vi "Qudi_multicolour_scan.vi"(3 "N Z positions":i32) -> ()   [LabVIEW 2015]
uses:
  <vilib>/rvi/Emulation/niFpgaGetClockAttributes.vi
  <vilib>/rvi/Emulation/niFpgaSctlEmulationGetInTimedLoop.vi
  <vilib>/rvi/Emulation/niFpgaEmulationReportErrorSimple.vi
  <vilib>/rvi/eio/common/nirviEmuTemplateMethod_errors.vi
  <vilib>/rvi/Emulation/niFpgaProcessEmulError.vi
  <vilib>/rvi/Emulation/niFpgaCriticalErrorInLSC.vi
  <vilib>/eio/EIONode/EIONode.xnode
panel:
  in  "exposure_time_ms":u16
  in  "stop":bool
  out "n cycles":i32
  out "Images acquired":i32
  in  "Laser lines":i32[](array[numeric])=[0, 0, 0, 0, 0, 0, 0, 0, 0, 0]
  in  "N laser lines":i32
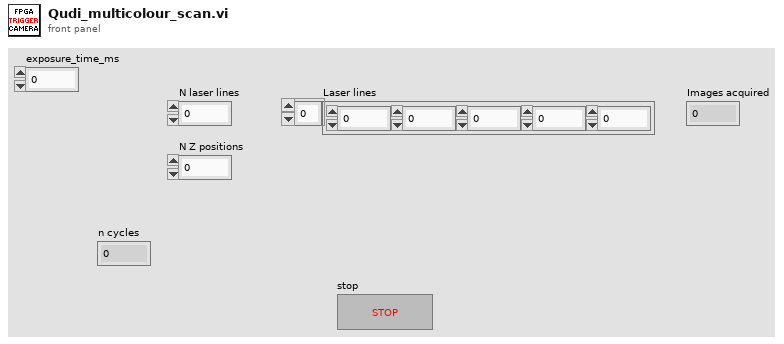
[diagram p1: front panel]
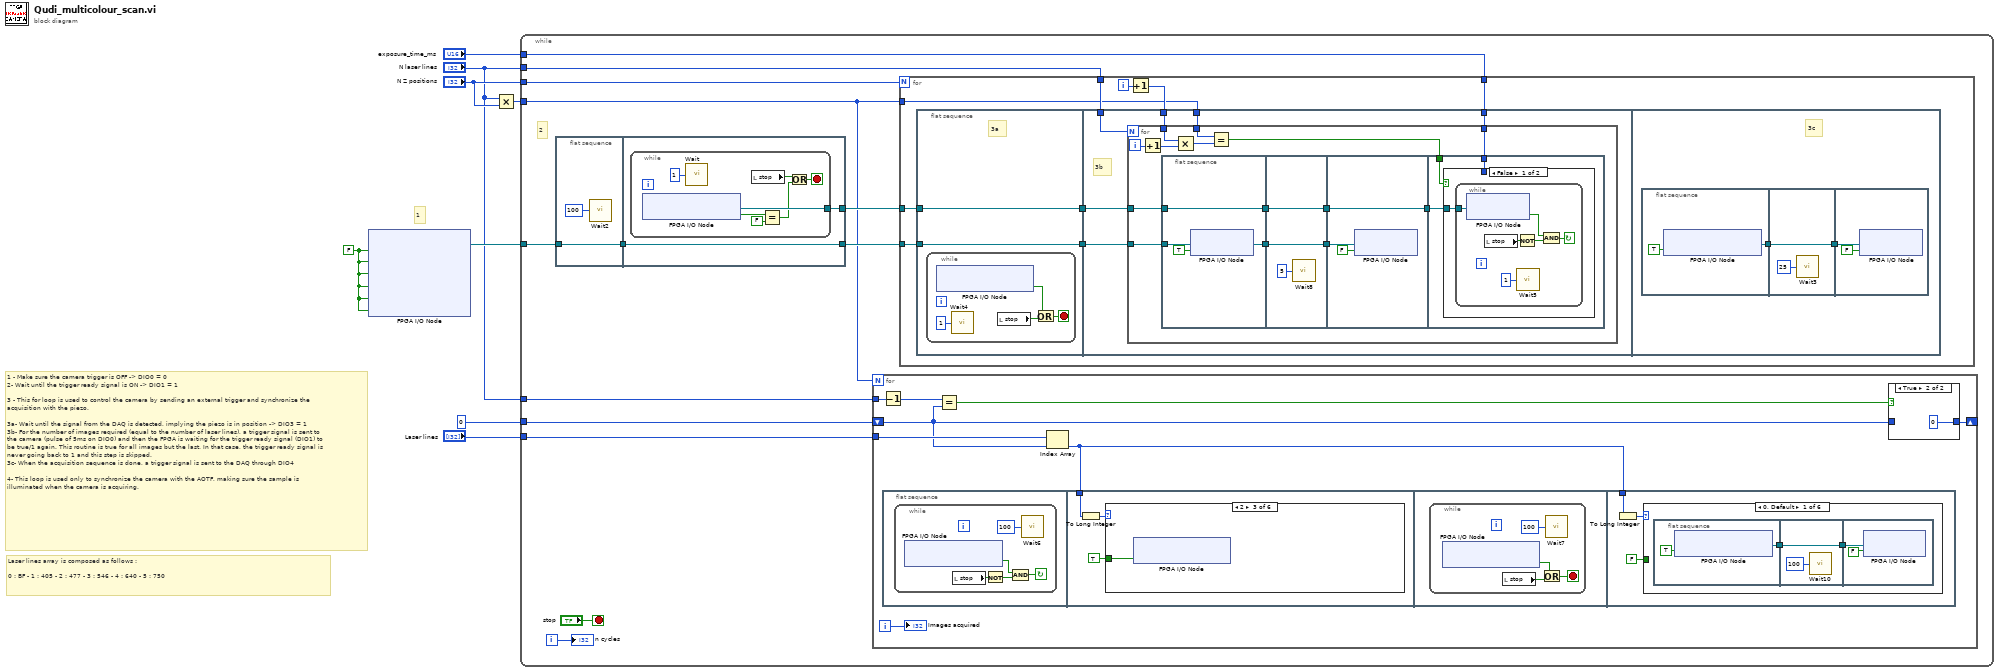
[diagram p0: block diagram]
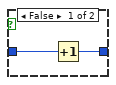
[diagram p2: hidden frame]
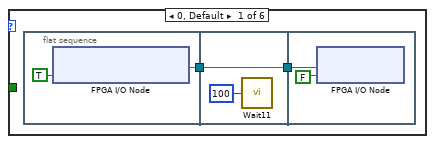
[diagram p3: hidden frame]
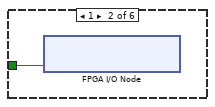
[diagram p4: hidden frame]
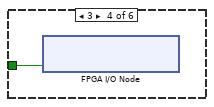
[diagram p5: hidden frame]
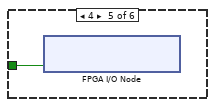
[diagram p6: hidden frame]
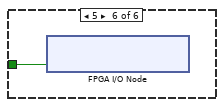
[diagram p7: hidden frame]
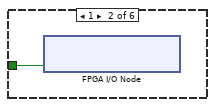
[diagram p8: hidden frame]
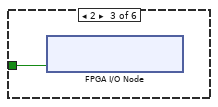
[diagram p9: hidden frame]
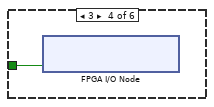
[diagram p10: hidden frame]
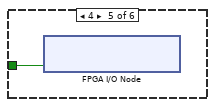
[diagram p11: hidden frame]
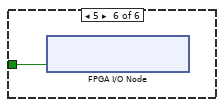
[diagram p12: hidden frame]
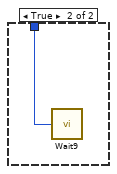
[diagram p13: hidden frame]
diagram:
  w1 = FALSE ("Connector0/DIO0")
  # "Laser lines array is composed as follows :\n\n0 : BF - 1 : 405 - 2 : 477 - 3 : 546 - 4 : 640 - 5 : 750"
  # "1"
  # "1 - Make sure the camera trigger is OFF -> DIO0 = 0\n2- Wait until the trigger ready signal is ON -> DIO1 = 1\n\n3 - This for loop is used to control the camera by sending an external trigger and synchronize the acquisition with the piezo.\n\n3a- Wait until the signal from the DAQ is detected, implying the piezo is in position -> DIO3 = 1 \n3b- For the number of images required (equal to the number of laser lines), a trigger signal is sent to the camera (pulse of 5ms on DIO0) and then the FPGA is waiting for the trigger ready signal (DIO1) to be true/1 again. This routine is true for all images but the last. In that case, the trigger ready signal is never going back to 1 and this step is skipped. \n3c- When the acquisition sequence is done, a trigger signal is sent to the DAQ through DIO4\n\n4- This loop is used only to synchronize the camera with the AOTF, making sure the sample is illuminated when the camera is acquiring."
  n1 = xnode "FPGA I/O Node"("Connector0/DIO0"=w1, "Connector0/DIO6"=w1, "Connector0/DIO7"=w1, "Connector0/DIO8"=w1, "Connector0/DIO9"=w1, "Connector0/DIO10"=w1) -> ("FPGA I/O Out"=w8:refnum<k21>)  [unwired: 6 in, 5 out]
  n2 = Multiply(x="N laser lines", y="N Z positions") -> (x*y=w4:i32)
  n3 = while {
    tunnel: w8 -> [w20]
    tunnel: "Laser lines" -> [w17]
    tunnel: 0 -> [w16]
    tunnel: "N Z positions" -> [w15]
    tunnel: "N laser lines" -> [w13]
    tunnel: w4 -> [w12]
    tunnel: "N laser lines" -> [w11]
    tunnel: "exposure_time_ms" -> [w10]
    i -> [w14]
    stop <- "stop" stop-if-true
    # "2"
    n4 = flat-sequence {
      tunnel: w20 -> [w75]
      tunnel: [w75] -> w21
      tunnel: w21 -> [w77]
      tunnel: [w77] -> w19
      tunnel: [w76] -> w18
      frame #0 {
        n5 = call "Wait2"("Count(uSec)"=u8 100 ("Count(mSec)")) -> ()  [unwired: 1 out]
      }
      frame #1 {
        n6 = while {
          tunnel: [w84] -> w76
          stop <- w79 stop-if-true
          n7 = xnode "FPGA I/O Node"() -> ("Connector0/DIO1"=w83:bool, "FPGA I/O Out"=w84:refnum<k21>)  [unwired: 1 in]
          n8 = call "Wait"("Count(mSec)"=u8 1) -> ()  [unwired: 1 out]
          n9 = local read "stop"() -> (w80:bool)
          n10 = Equal?(x=w83, y=FALSE) -> (x = y?=w81:bool)
          n11 = Or(x=w80, y=w81) -> (x .or. y?=w79:bool)
        }
      }
    }
    n12 = for {
      N: w12 -> [_]
      shift-right: [w27] -> _
      shift-left: w16 -> [w25]
      tunnel: w17 -> [w26]
      tunnel: w11 -> [w24]
      i -> [w22]
      n13 = Decrement(x=w24) -> (x-1=w23:i32)
      n14 = flat-sequence {
        tunnel: w29 -> [w39]
        tunnel: w29 -> [w58]
        frame #0 {
          n15 = while {
            stop <- w34 continue-if-true
            n16 = xnode "FPGA I/O Node"() -> ("Connector0/DIO2"=w35:bool)  [unwired: 1 in, 1 out]
            n17 = local read "stop"() -> (w36:bool)
            n18 = Not(x=w36) -> (.not. x?=w37:bool)
            n19 = And(x=w35, y=w37) -> (x .and. y?=w34:bool)
            n20 = call "Wait6"("Count(uSec)"=u8 100 ("Count(mSec)")) -> ()  [unwired: 1 out]
          }
        }
        frame #1 {
          n21 = To Long Integer(number=w39) -> (32bit integer=w40:i32)
          n22 = case shown="2" w40 {
            tunnel: TRUE ("Connector0/DIO6") -> [_ w49 w50 w51 w52 w53]
            frame 0, Default {
              n23 = flat-sequence {
                tunnel: [w43] -> w42
                tunnel: w42 -> [w45]
                tunnel: [w45] -> w41
                tunnel: w41 -> [w48]
                frame #0 {
                  n24 = xnode "FPGA I/O Node"("Connector0/DIO5"=TRUE) -> ("FPGA I/O Out"=w43:refnum<k21>)  [unwired: 1 in]
                }
                frame #1 {
                  n25 = call "Wait11"("Count(uSec)"=u32 100) -> ()  [unwired: 1 out]
                }
                frame #2 {
                  n26 = xnode "FPGA I/O Node"("I/O Item"=FALSE, "FPGA I/O In"=w48) -> ()  [unwired: 1 out]
                }
              }
            }
            frame 1 {
              n27 = xnode "FPGA I/O Node"("Connector0/DIO8"=w49) -> ()  [unwired: 1 in, 1 out]
            }
            frame 2 {
              n28 = xnode "FPGA I/O Node"("Connector0/DIO9"=w50) -> ()  [unwired: 1 in, 1 out]
            }
            frame 3 {
              n29 = xnode "FPGA I/O Node"("Connector0/DIO6"=w51) -> ()  [unwired: 1 in, 1 out]
            }
            frame 4 {
              n30 = xnode "FPGA I/O Node"("Connector0/DIO7"=w52) -> ()  [unwired: 1 in, 1 out]
            }
            frame 5 {
              n31 = xnode "FPGA I/O Node"("Connector0/DIO10"=w53) -> ()  [unwired: 1 in, 1 out]
            }
          }
        }
        frame #2 {
          n32 = while {
            stop <- w55 stop-if-true
            n33 = xnode "FPGA I/O Node"() -> ("Connector0/DIO2"=w56:bool)  [unwired: 1 in, 1 out]
            n34 = local read "stop"() -> (w57:bool)
            n35 = Or(x=w56, y=w57) -> (x .or. y?=w55:bool)
            n36 = call "Wait7"("Count(uSec)"=u8 100 ("Count(mSec)")) -> ()  [unwired: 1 out]
          }
        }
        frame #3 {
          n37 = To Long Integer(number=w58) -> (32bit integer=w59:i32)
          n38 = case shown="0, Default" w59 {
            tunnel: FALSE ("Connector0/DIO6") -> [_ w69 w70 w71 w72 w73]
            frame 0, Default {
              n39 = flat-sequence {
                tunnel: [w63] -> w62
                tunnel: w62 -> [w65]
                tunnel: [w65] -> w61
                tunnel: w61 -> [w68]
                frame #0 {
                  n40 = xnode "FPGA I/O Node"("Connector0/DIO5"=TRUE) -> ("FPGA I/O Out"=w63:refnum<k21>)  [unwired: 1 in]
                }
                frame #1 {
                  n41 = call "Wait10"("Count(uSec)"=u32 100) -> ()  [unwired: 1 out]
                }
                frame #2 {
                  n42 = xnode "FPGA I/O Node"("I/O Item"=FALSE, "FPGA I/O In"=w68) -> ()  [unwired: 1 out]
                }
              }
            }
            frame 1 {
              n43 = xnode "FPGA I/O Node"("Connector0/DIO8"=w69) -> ()  [unwired: 1 in, 1 out]
            }
            frame 2 {
              n44 = xnode "FPGA I/O Node"("Connector0/DIO9"=w70) -> ()  [unwired: 1 in, 1 out]
            }
            frame 3 {
              n45 = xnode "FPGA I/O Node"("Connector0/DIO6"=w71) -> ()  [unwired: 1 in, 1 out]
            }
            frame 4 {
              n46 = xnode "FPGA I/O Node"("Connector0/DIO7"=w72) -> ()  [unwired: 1 in, 1 out]
            }
            frame 5 {
              n47 = xnode "FPGA I/O Node"("Connector0/DIO10"=w73) -> ()  [unwired: 1 in, 1 out]
            }
          }
        }
      }
      n48 = Equal?(x=w23, y=w25) -> (x = y?=w28:bool)
      n49 = Index Array(array=w26, index=w25) -> (element=w29:i32)
      n50 = case shown="True" w28 {
        tunnel: w25 -> [w31 _]
        tunnel: [w30 0] -> w27
        frame False {
          n51 = Increment(x=w31) -> (x+1=w30:i32)
        }
        frame True {
        }
      }
      "Images acquired" <- w22
    }
    n52 = for {
      N: w15 -> [_]
      tunnel: w19 -> [w92]
      tunnel: w18 -> [w93]
      tunnel: w13 -> [w88]
      tunnel: w12 -> [w86]
      tunnel: w10 -> [w85]
      i -> [w89]
      n53 = flat-sequence {
        tunnel: w92 -> [w94]
        tunnel: w93 -> [w95]
        tunnel: [w95] -> w91
        tunnel: [w94] -> w90
        tunnel: w91 -> [w105]
        tunnel: w90 -> [w104]
        tunnel: w88 -> [w103]
        tunnel: w87 -> [w102]
        tunnel: w86 -> [w101]
        tunnel: w85 -> [w100]
        frame #0 {
          # "3a"
          n54 = while {
            stop <- w97 stop-if-true
            n55 = xnode "FPGA I/O Node"() -> ("Connector0/DIO3"=w98:bool)  [unwired: 1 in, 1 out]
            n56 = call "Wait4"("Count(mSec)"=u8 1) -> ()  [unwired: 1 out]
            n57 = local read "stop"() -> (w99:bool)
            n58 = Or(x=w98, y=w99) -> (x .or. y?=w97:bool)
          }
        }
        frame #1 {
          # "3b"
          n59 = for {
            N: w103 -> [_]
            tunnel: w105 -> [w114]
            tunnel: w104 -> [w113]
            tunnel: w102 -> [w110]
            tunnel: w101 -> [w108]
            tunnel: w100 -> [w106]
            i -> [w112]
            n60 = Increment(x=w112) -> (x+1=w111:i32)
            n61 = flat-sequence {
              tunnel: [w122] -> w119
              tunnel: [w120] -> w118
              tunnel: w113 -> [w121]
              tunnel: w114 -> [w120]
              tunnel: w119 -> [w126]
              tunnel: [w126] -> w117
              tunnel: [w125] -> w116
              tunnel: w118 -> [w125]
              tunnel: w117 -> [w128]
              tunnel: [w127] -> w115
              tunnel: w116 -> [w127]
              tunnel: w115 -> [w132]
              tunnel: w107 -> [w131]
              tunnel: w106 -> [w130]
              frame #0 {
                n62 = xnode "FPGA I/O Node"("I/O Item"=TRUE ("Connector0/DIO0"), "FPGA I/O In"=w121) -> ("FPGA I/O Out"=w122:refnum<k21>)
              }
              frame #1 {
                n63 = call "Wait8"("Count(mSec)"=u8 5) -> ()  [unwired: 1 out]
              }
              frame #2 {
                n64 = xnode "FPGA I/O Node"("I/O Item"=FALSE ("Connector0/DIO0"), "FPGA I/O In"=w128) -> ()  [unwired: 1 out]
              }
              frame #3 {
                n65 = case shown="False" w131 {
                  tunnel: w132 -> [w133 _]
                  tunnel: w130 -> [_ w140]
                  frame False {
                    n66 = while {
                      tunnel: w133 -> [w139]
                      stop <- w135 continue-if-true
                      n67 = xnode "FPGA I/O Node"("FPGA I/O In"=w139) -> ("I/O Item"=w136:bool)  [unwired: 1 out]
                      n68 = local read "stop"() -> (w138:bool)
                      n69 = Not(x=w138) -> (.not. x?=w137:bool)
                      n70 = call "Wait5"("Count(mSec)"=u8 1) -> ()  [unwired: 1 out]
                      n71 = And(x=w136, y=w137) -> (x .and. y?=w135:bool)
                    }
                  }
                  frame True {
                    n72 = call "Wait9"("Count(mSec)"=w140) -> ()  [unwired: 1 out]
                  }
                }
              }
            }
            n73 = Multiply(x=w110, y=w111) -> (x*y=w109:i32)
            n74 = Equal?(x=w108, y=w109) -> (x = y?=w107:bool)
          }
        }
        frame #2 {
          # "3c"
          n75 = flat-sequence {
            tunnel: [w144] -> w142
            tunnel: w142 -> [w145]
            tunnel: [w145] -> w141
            tunnel: w141 -> [w147]
            frame #0 {
              n76 = xnode "FPGA I/O Node"("Connector0/DIO4"=TRUE) -> ("FPGA I/O Out"=w144:refnum<k21>)  [unwired: 1 in]
            }
            frame #1 {
              n77 = call "Wait3"("Count(mSec)"=u8 25) -> ()  [unwired: 1 out]
            }
            frame #2 {
              n78 = xnode "FPGA I/O Node"("I/O Item"=FALSE ("Connector0/DIO0"), "FPGA I/O In"=w147) -> ()  [unwired: 1 out]
            }
          }
        }
      }
      n79 = Increment(x=w89) -> (x+1=w87:i32)
    }
    "n cycles" <- w14
  }
